vi "exportLvDll.vi"(11 "count":i32) -> (3 "outArray":dbl[](array[numeric]))   [LabVIEW 2020]
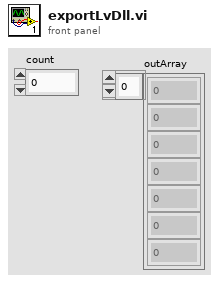
[diagram p1: front panel]
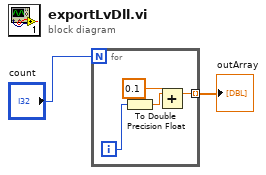
[diagram p0: block diagram]
diagram:
  n1 = for {
    N: "count" -> [_]
    tunnel: [w4] -> w1 mode=indexing
    i -> [w6]
    n2 = To Double Precision Float(number=w6) -> (double precision float=w5:dbl)
    n3 = Add(x=w5, y=0.1) -> (x+y=w4:dbl)
  }
  "outArray" <- w1
